vi "Data To Dashboard.vi"(0 "Viewer Select":T1(ring)=enum."Ball Camera", 1 "Hoop Select":T2(ring), 2 "Number Of Balls":i32, 3 "Shooting Manual Override?":bool, 4 "Ball Managment Manual Override?":bool, 5 "Error!":bool, 6 "Engaging Manual Override?":bool, 7 "Aligning?":bool, 8 "Bridge Mode?":bool, 9 "Right Side":bool, 10 "Tank?":bool, 11 "Collecting Balls?":bool, 12 "Aligned?":bool, 13 "Repelling Balls?":bool, 14 "Shooter Is front":bool) -> ()   [LabVIEW 2011]
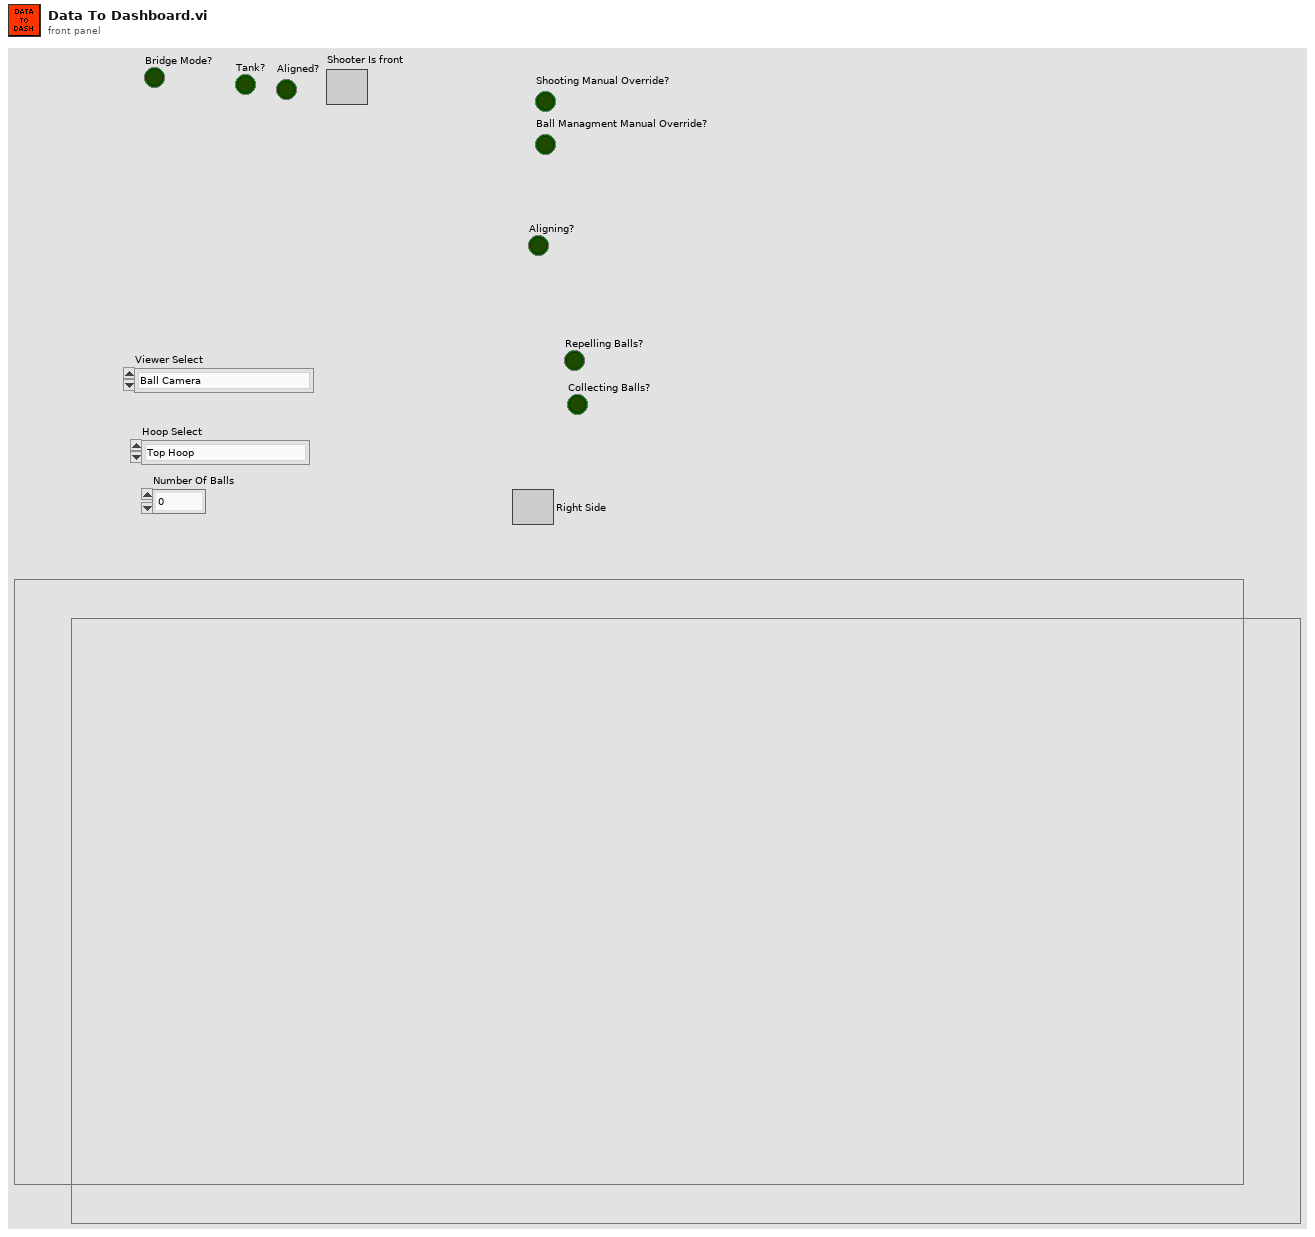
[diagram p1: front panel]
types:
  T1 = enum32{"Target Camera", "Target Camera Mask", "Ball Camera", "Kinect Skeleton"}
  T2 = enum32{"Top Hoop", "Bottom Hoop", "Left Hoop", "Right Hoop"}
  T3 = cluster{"Viewer Select":enum32{"Target Camera", "Target Camera Mask", "Ball Camera", "Kinect Skeleton"}, "Hoop Select":enum32{"Top Hoop", "Bottom Hoop", "Left Hoop", "Right Hoop"}, "Flashy the LED":bool, "Number Of Balls":i32, "Tank?":bool, "Bridge Mode?":bool, "Shooting Manual Override?":bool, "Ball Managment Manual Override?":bool, "Error!":bool, "Engaging Manual Override?":bool, "Shooter Is front  ":bool, "Right Side":bool, "Repelling Balls?":bool, "Collecting Balls?":bool}
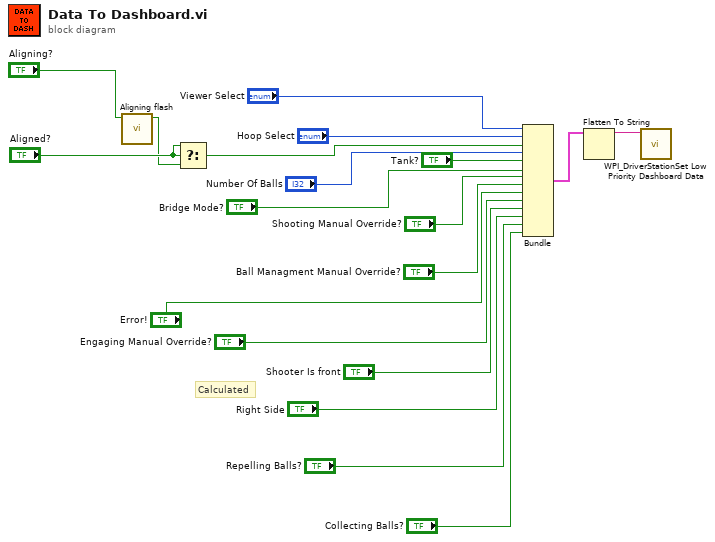
[diagram p0: block diagram]
diagram:
  # "Calculated"
  n1 = call "Aligning flash.vi"("Thing 1"="Aligning?") -> ("Flashy the LED"=w7:bool)  [unwired: 10 in]
  n2 = Select(t="Aligned?", s="Aligned?", f=w7) -> (s? t:f=w5:bool)
  n3 = Bundle("Viewer Select"="Viewer Select", "Hoop Select"="Hoop Select", "Flashy the LED"=w5, "Number Of Balls"="Number Of Balls", "Tank?"="Tank?", "Bridge Mode?"="Bridge Mode?", "Shooting Manual Override?"="Shooting Manual Override?", "Ball Managment Manual Override?"="Ball Managment Manual Override?", "Error!"="Error!", "Engaging Manual Override?"="Engaging Manual Override?", "Shooter Is front"="Shooter Is front", "Right Side"="Right Side", "Repelling Balls?"="Repelling Balls?", "Collecting Balls?"="Collecting Balls?") -> (w19:T3)  [unwired: 1 in]
  n4 = Flatten To String(anything=w19) -> (data string=w18:string)  [unwired: 3 in, 2 out]
  n5 = call <vilib>:"WPI_DriverStationSet Low Priority Dashboard Data.vi"("User Data"=w18) -> ()  [unwired: 10 in, 1 out]
